vi "Fpga-OrderBook.vi"() -> ()   [LabVIEW 2016]
uses:
  <vilib>/Platform/TimedLoop/XDataNode/timing_clust.ctl
  <vilib>/Platform/TimedLoop/XDataNode/nitl_modes.ctl
  <vilib>/Platform/TimedLoop/XDataNode/wakeup.ctl
  <vilib>/rvi/Emulation/niFpgaSctlEmulationGetInTimedLoop.vi
  <vilib>/rvi/Emulation/niFpgaEmulationReportErrorSimple.vi
  <vilib>/rvi/Emulation/niFpgaGetClockAttributes.vi
  <vilib>/rvi/Emulation/niFpgaCriticalErrorInLSC.vi
  <vilib>/rvi/DataTransferAndStorage/Container/Common/niFpgaContainerGetUniqueNameForEmu.vi
  <vilib>/rvi/DataTransferAndStorage/Container/Common/niFpgaContainerSetEmuInfo.vi
  <vilib>/rvi/eio/common/nirviEmuReportErrorAndStop.vi
  <vilib>/rvi/DataTransferAndStorage/Container/Common/niFpgaContainerExecOnDevCompGetState.vi
  <vilib>/rvi/Emulation/niFpgaEmulationIsFPGAContextNoSignature.vi
  <vilib>/rvi/Emulation/niFpgaProcessEmulError.vi
  <vilib>/rvi/errors/nirviReportUnexpectedCaseInternalError (U32).vi
  <vilib>/rvi/Memory/Memory_Emulation/niFpgaMemoryEmulationCacheClearOnFirstRun.vi
  <vilib>/rvi/Memory/Memory_Emulation/nirvimemoryEmulationManagerCache_MakeExclusive.vi
  <vilib>/rvi/Memory/Memory_Emulation/niFpgaMemoryEmulationValidateCache.vi
  <vilib>/rvi/Memory/Memory_Emulation/nirvimemoryEmulationManagerCache_InsertValue.vi
  <vilib>/Utility/error.llb/Clear Errors.vi
  <vilib>/rvi/Memory/Memory_Emulation/nirvimemoryEmulationManagerCache_ReleaseExclusive.vi
  <vilib>/rvi/Memory/Memory_Emulation/nirvimemoryEmulationManagerCache_GetValue.vi
  <vilib>/rvi/Memory/Memory_Emulation/nirvimemoryEmulationManagerCache_SetValue.vi
  <vilib>/rvi/Emulation/niFpgaSctlEmulationResourceMgr.vi
  <vilib>/rvi/errors/niFpgaSetErrorForExecOnDevCompSimple.vi
  <vilib>/rvi/FIFO/Fifo_Resource/nirvififoEmulationSetSize.vi
  <vilib>/rvi/FIFO/Fifo_Resource/nirviFifoEmulationQueueMgr.vi
  <instcachedir>/0/nirviFifoEmulationQueueMgr_E5CAEC123FF24DC58D834DCA3CDAA9B5.lvgen/nirviFifoEmulationQueueMgr_E5CAEC123FF24DC58D834DCA3CDAA9B5_000.vi
  <vilib>/rvi/FIFO/Fifo_Resource/nirvififoEmulationDetermineInputValidOut.vi
  <vilib>/rvi/FIFO/Fifo_Resource/nirvififoEmulationCreateLock.vi
  <vilib>/rvi/FIFO/Fifo_Resource/nirvififoEmulationObtainLock.vi
  <vilib>/rvi/FIFO/Fifo_Resource/nirvififoEmulationReleaseLock.vi
  <vilib>/rvi/occurrence/nirviWaitOnOccurrenceBase.vi
  <vilib>/rvi/errors/nirviReportUnexpectedCaseInternalError.vi
  <vilib>/Platform/TimedLoop/XDataNode/XDataNode.xnode
  <vilib>/rvi/LocalResourceManager/LocalResourceManager.xnode
  <vilib>/rvi/DataTransferAndStorage/Container/XNode/niFpgaContainer.xnode
  <vilib>/rvi/Memory/Memory_Emulation/niFpgaMemoryEmulationRefIn.vi
  <vilib>/rvi/FIFO/Fifo_Resource/nirvififoEmulationWrite.vi
  <vilib>/rvi/FIFO/Fifo_Resource/nirvififoEmulationRead.vi
  <vilib>/Platform/TimedLoop/XDataNode/XDNodeRunTimeDep.lvlib
panel:
  out "Command being Read":bool
  out "Command":T1 {"OrderRefNum" format="%.0x"}
  out "Command\nExecuting":bool
  out "Counter":u64 format="%.0x"
  out "Command":u16 format="%.0x"
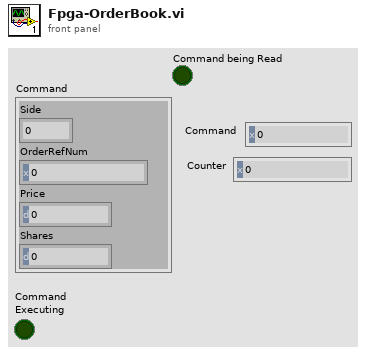
[diagram p1: front panel]
types:
  T1 = cluster{"Side":u16, "OrderRefNum":u64, "Price":u32, "Shares":u32}
  T2 = typedef "XDNodeRunTimeDep.lvlib/timing_clust.ctl" = cluster{"Expected End [f-1]":u64, "Actual End [f-1]":u64, "Finished Late? [f-1]":bool, "Expected End [i-1]":u64, "Actual End [i-1]":u64, "Finished Late? [i-1]":bool, "Expected Start [i]":u64, "Actual Start [i]":u64, "Expected Start [f]":u64, "Actual Start [f]":u64, "Source Name":string, "Structure Name":string, "Period":i64, "Deadline":i64, "Offset":i64, "Start":i64, "Priority":i32, "Timeout":i32, "Mode":T3, "Wakeup Reason":T4, "Error":errorcluster, "Source Type":string, "Secondary Source Type":string, "Global End Time":u64, "Global Start Time":u64, "Frame Duration":u64, "Iteration Duration":u64, "Assigned CPU":i32, "I/O Scan Engine Mode":u32}
  T3 = typedef "XDNodeRunTimeDep.lvlib/nitl_modes.ctl" = enum32{"No Change", "Process missed periods, maintain original phase", "Discard missed periods, maintain original phase", "Process missed periods, ignore original phase", "Discard missed periods, ignore original phase"}
  T4 = typedef "XDNodeRunTimeDep.lvlib/wakeup.ctl" = enum32{"Normal", "Aborted", "Asynchronous wakeup", "Timing source error", "Timed loop error", "Timeout"}
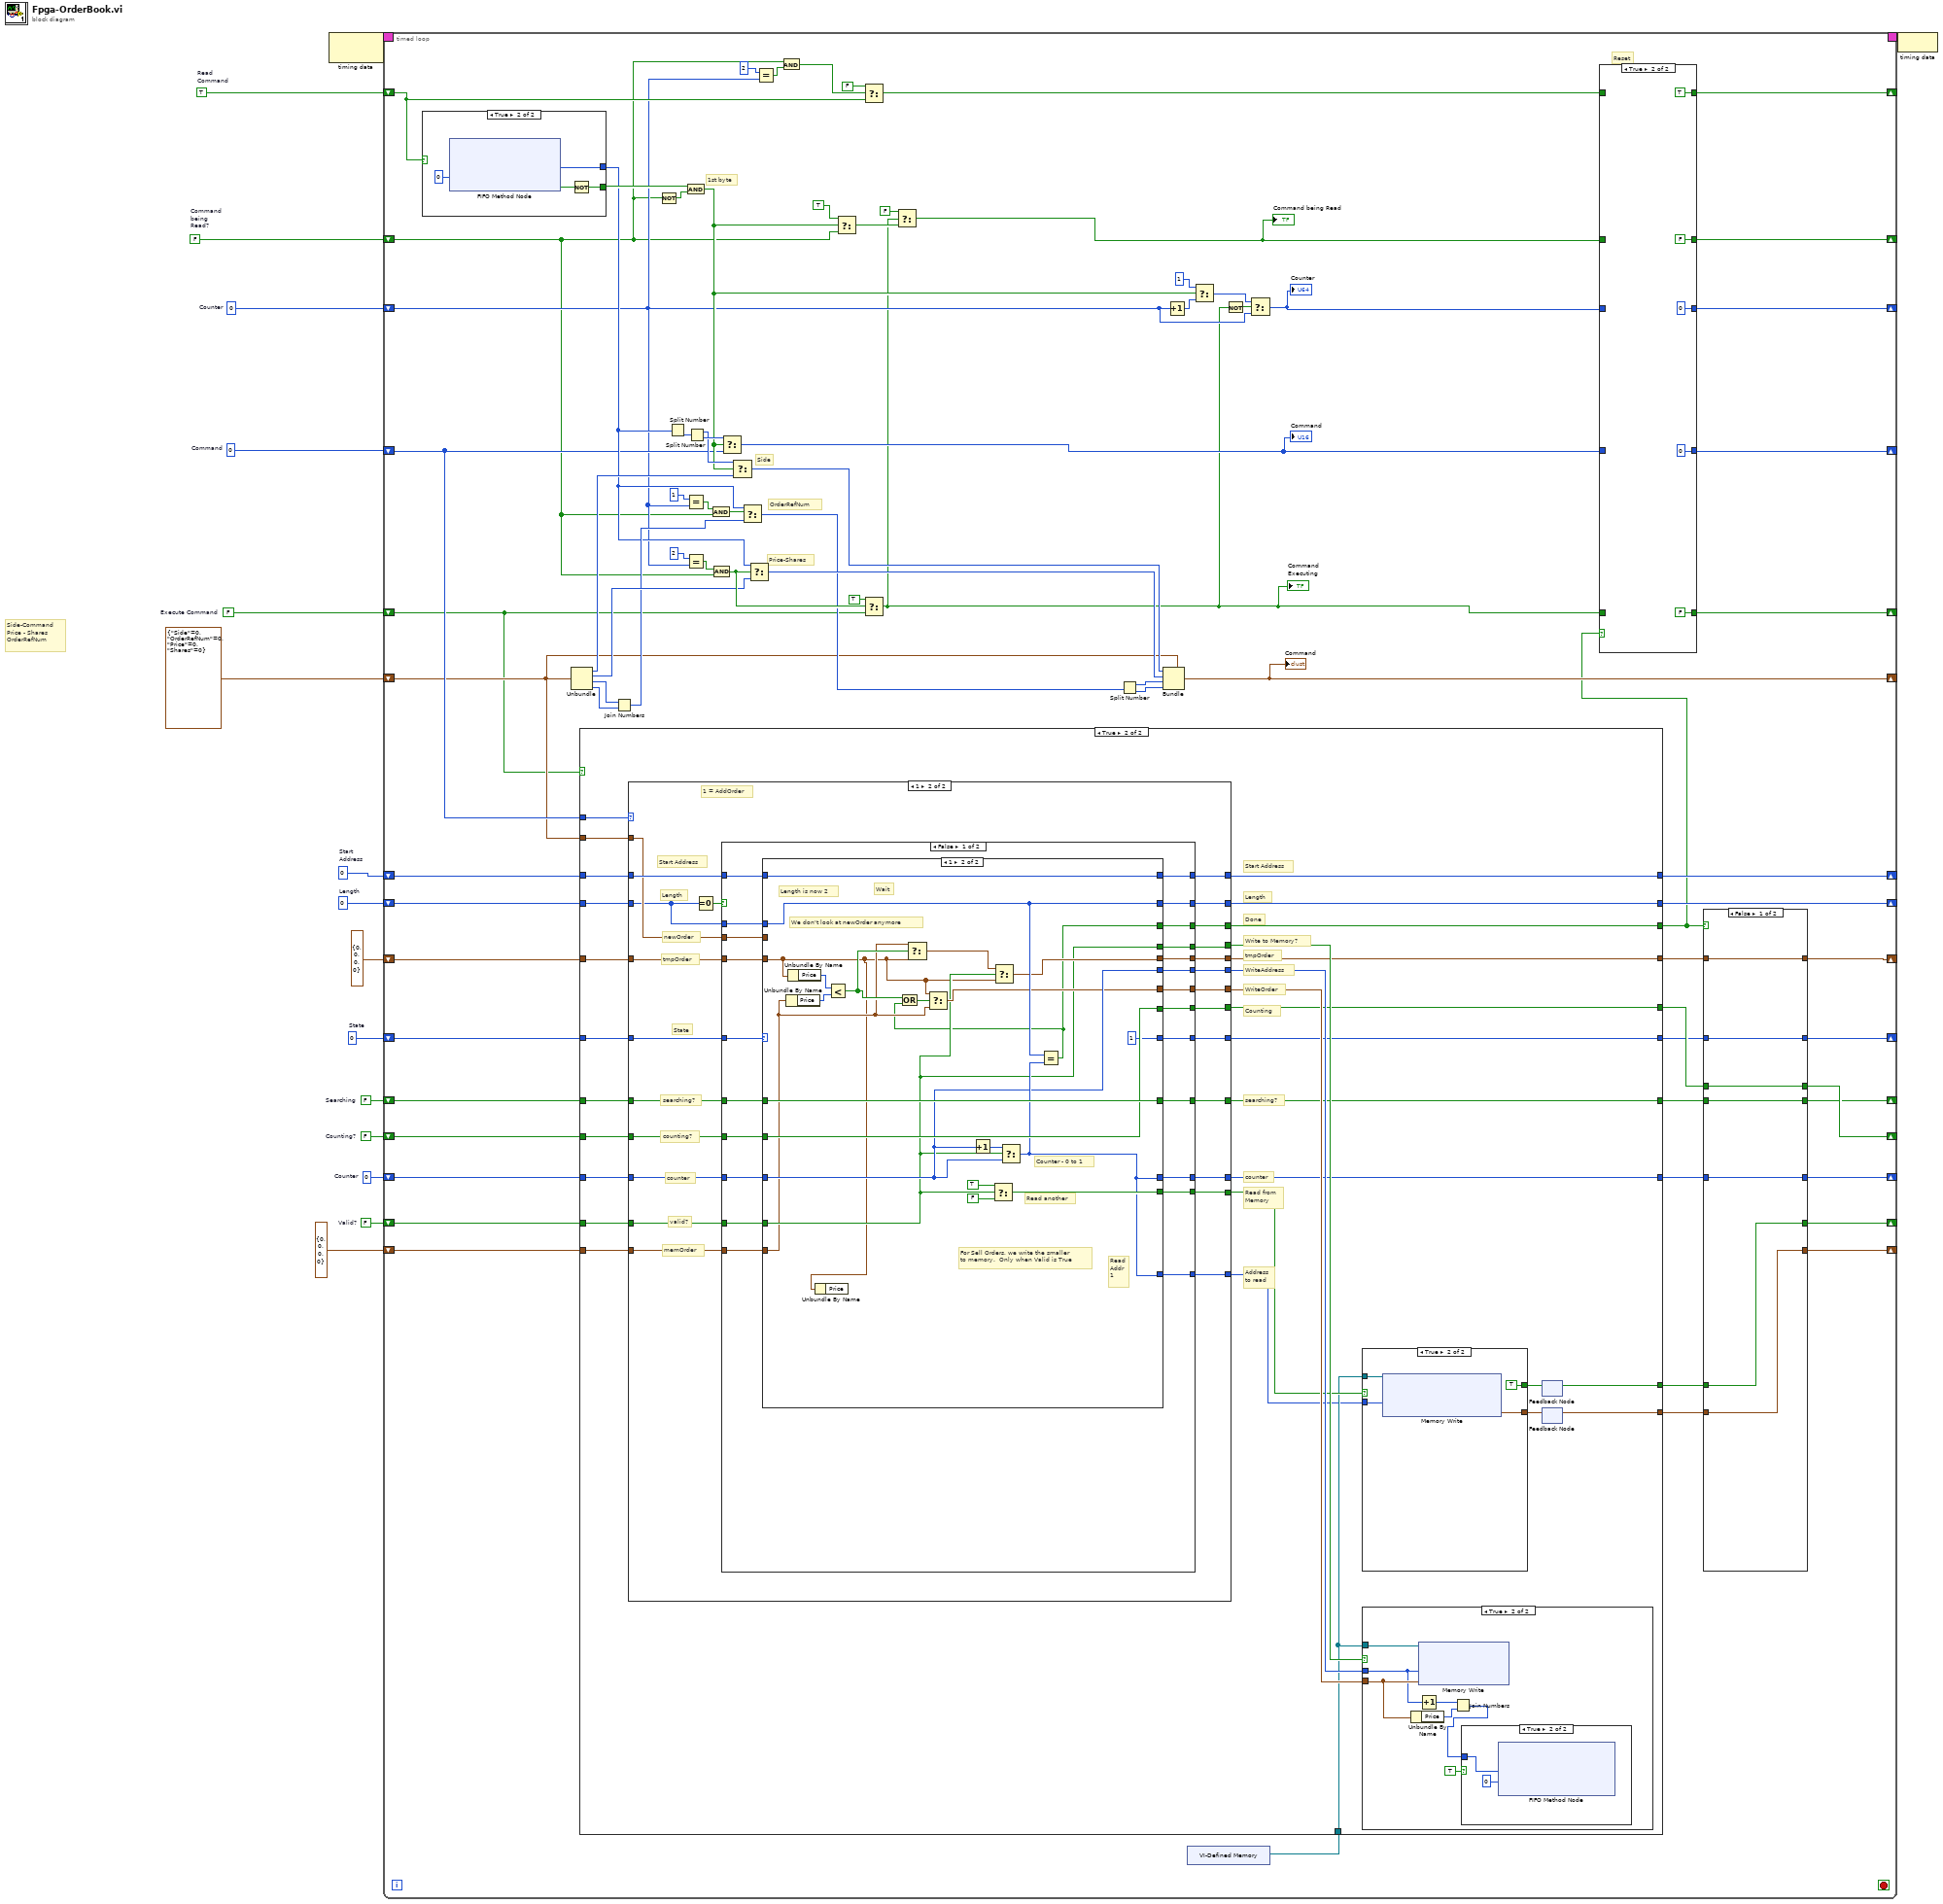
[diagram p0: block diagram]
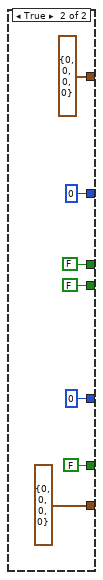
[diagram p2: hidden frame]
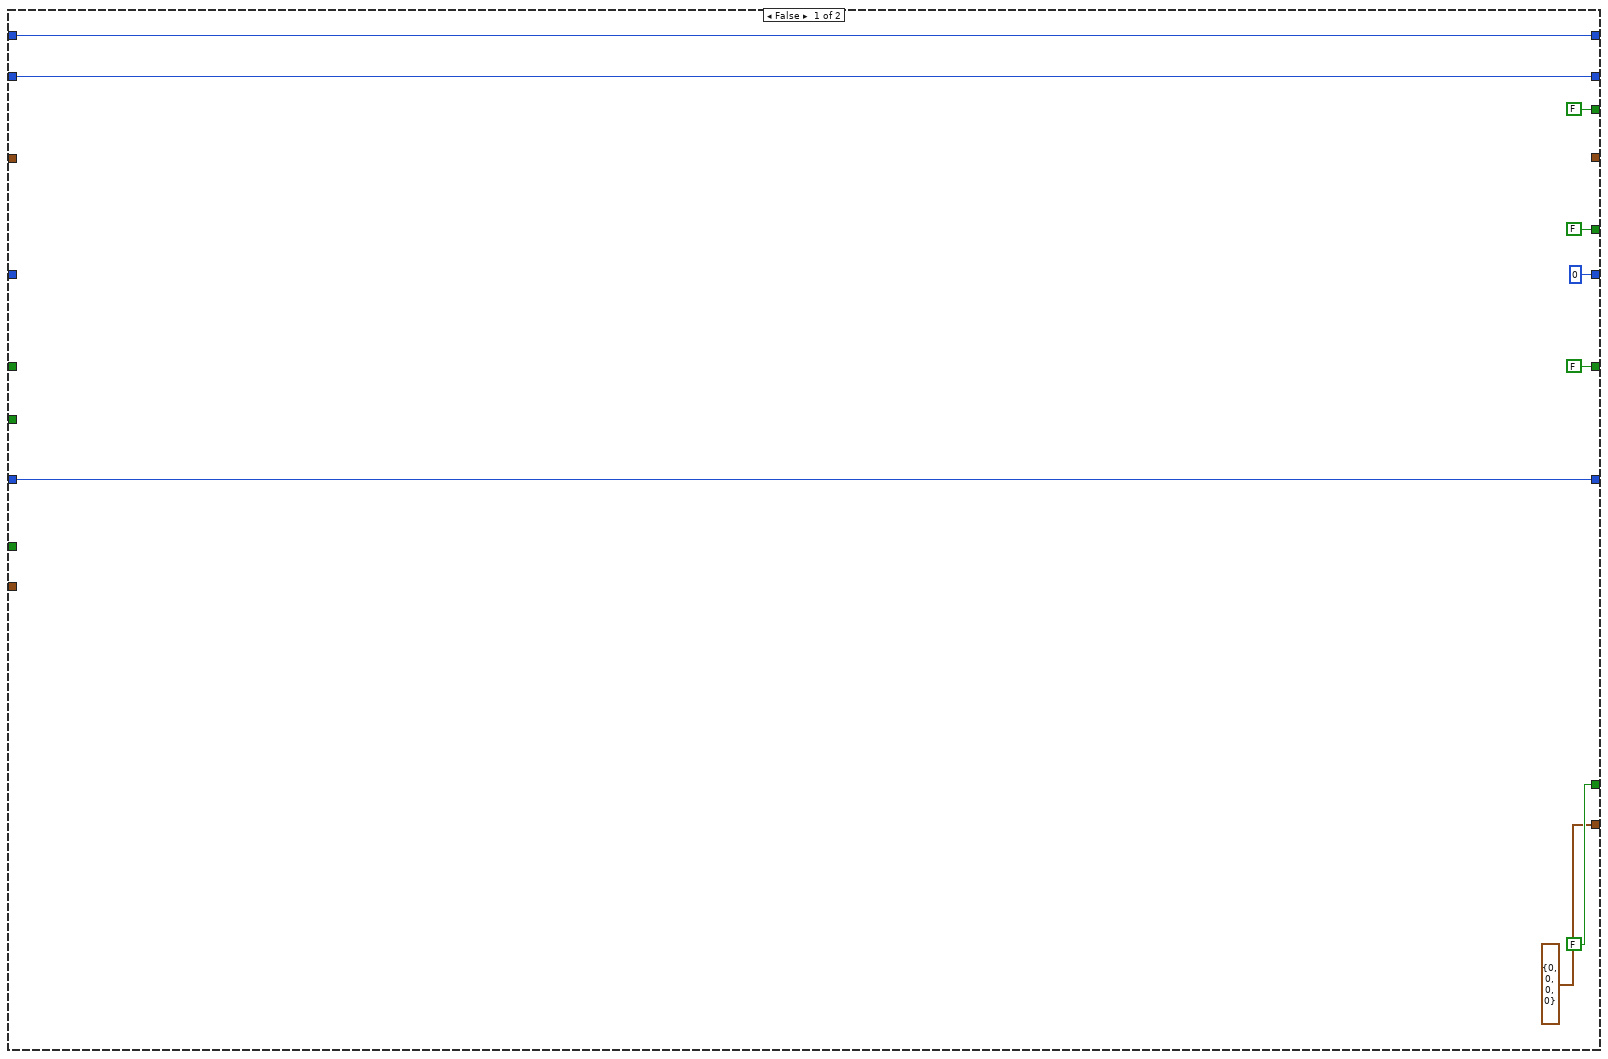
[diagram p4: hidden frame]
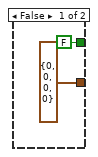
[diagram p5: hidden frame]
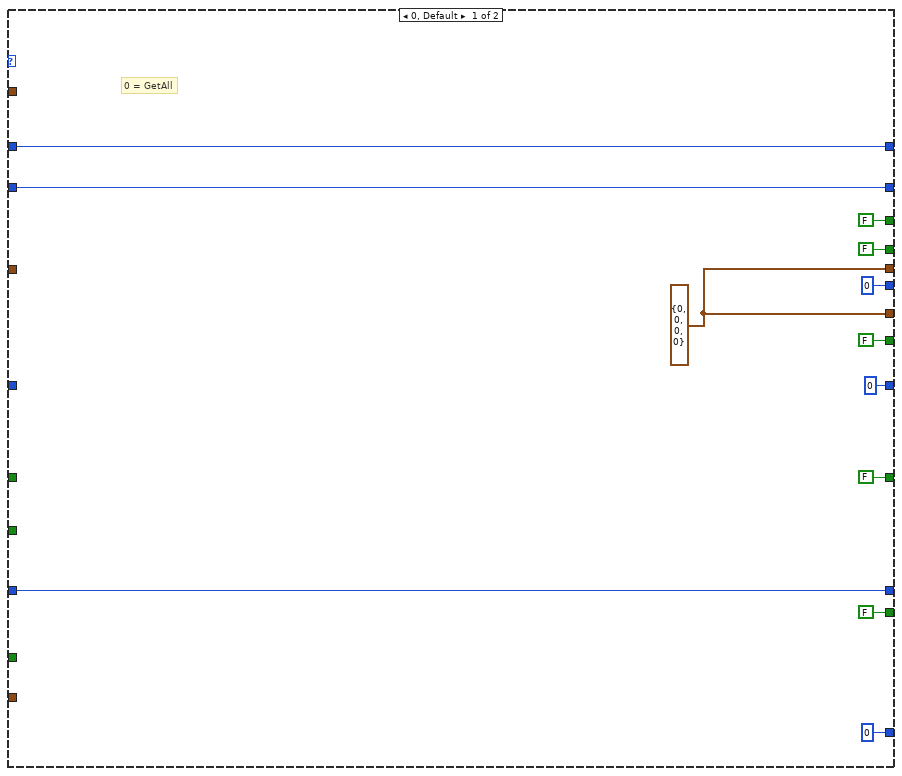
[diagram p8: hidden frame]
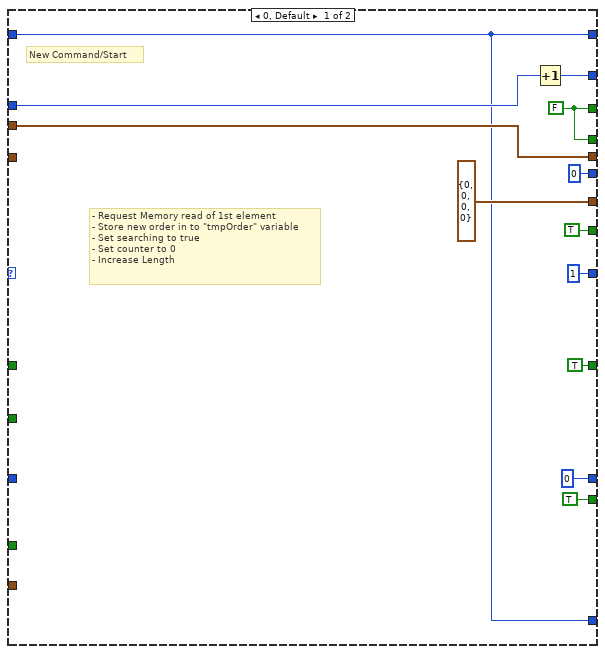
[diagram p9: hidden frame]
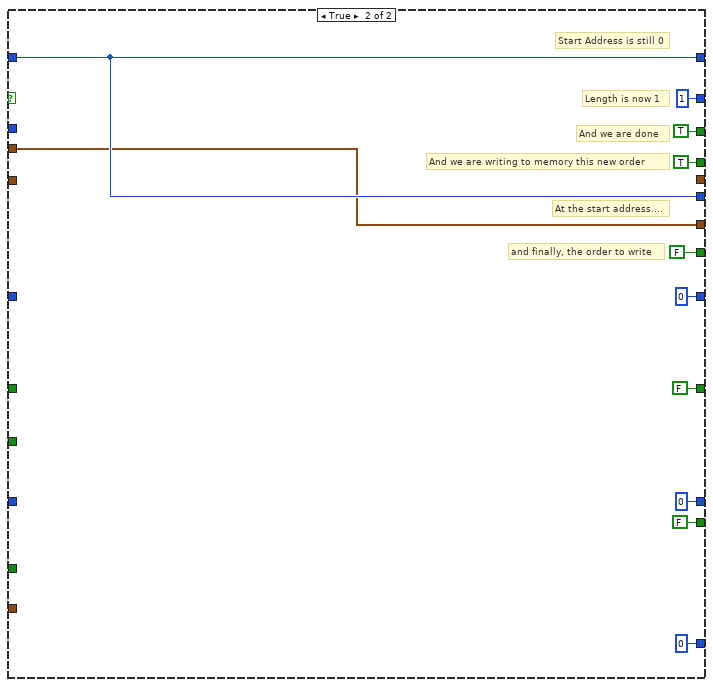
[diagram p10: hidden frame]
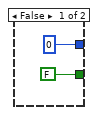
[diagram p11: hidden frame]
diagram:
  w1 = i16 0  # State
  w3 = FALSE  # Searching
  w5 = FALSE  # Valid?
  w6 = FALSE  # Counting?
  w8 = u64 0  # Counter
  w9 = FALSE  # Execute Command
  w11 = u64 0  # Length
  w10 = u64 0  # Start Address
  w12 = u64 0  # Counter
  w13 = u16 0  # Command
  w14 = FALSE  # Command being Read?
  w15 = TRUE  # Read Command
  # "Side-Command\nPrice - Shares\nOrderRefNum"
  n1 = node-c288() -> (w17:T2)  [unwired: 1 in]
  n2 = timed-loop {
    timing: w17 -> [_]
    timing-out: [_] -> w16
    shift-right: [w47] -> _
    shift-left: w15 -> [w93]
    shift-right: [w46] -> _
    shift-left: w14 -> [w51]
    shift-right: [w42] -> _
    shift-left: w13 -> [w58]
    shift-right: [w44] -> _
    shift-left: w12 -> [w55]
    shift-right: [w86] -> _
    shift-left: w10 -> [w87]
    shift-right: [w88] -> _
    shift-left: w11 -> [w89]
    shift-right: [w40] -> _
    shift-left: w9 -> [w49]
    shift-right: [w29] -> _
    shift-left: w8 -> [w79]
    shift-right: [w73] -> _
    shift-left: T1 {"Side"=0, "OrderRefNum"=0, "Price"=0, "Shares"=0} ("Cluster") -> [w50]
    shift-right: [w32] -> _
    shift-left: w6 -> [w38]
    shift-right: [w23] -> _
    shift-left: T1 {"Side"=0, "OrderRefNum"=0, "Price"=0, "Shares"=0} ("Data") -> [w36]
    shift-right: [w24] -> _
    shift-left: w5 -> [w37]
    shift-right: [w31] -> _
    shift-left: w3 -> [w35]
    shift-right: [w27] -> _
    shift-left: T1 {"Side"=0, "OrderRefNum"=0, "Price"=0, "Shares"=0} ("Data") -> [w34]
    shift-right: [w20] -> _
    shift-left: w1 -> [w21]
    stop <- _ stop-if-true
    # "Reset"
    # "Price-Shares"
    # "OrderRefNum"
    # "Side"
    # "1st byte"
    n3 = case shown="True" w93 {
      tunnel: [FALSE ("Timed Out?") w280] -> w95
      tunnel: [u64 0 ("Element") w281] -> w60
      frame False {
      }
      frame True {
        n4 = xnode ("FIFO Method Node")("Timeout"=0) -> ("Element"=w281:u64, "Timed Out?"=w282:bool)  [unwired: 1 in, 1 out]
        n5 = Not(x=w282) -> (.not. x?=w280:bool)
      }
    }
    n6 = Unbundle(w50) -> ("Side"=w63:u16, "OrderRefNum"=w70:u64, "Price"=w66:u32, "Shares"=w65:u32)
    n7 = Join Numbers(hi=w66, lo=w65) -> ((hi.lo)=w61:u64)
    n8 = Not(x=w51) -> (.not. x?=w96:bool)
    n9 = Split Number(x=w60) -> (lo(x)=w72:u32)  [unwired: 1 out]
    n10 = And(x=w95, y=w96) -> (x .and. y?=w59:bool)
    n11 = Equal?(x=u64 1, y=w55) -> (x = y?=w52:bool)
    n12 = Equal?(x=u64 2, y=w55) -> (x = y?=w77:bool)
    n13 = Split Number(x=w72) -> (hi(x)=w62:u16, lo(x)=w64:u16)
    n14 = And(x=w52, y=w51) -> (x .and. y?=w53:bool)
    n15 = And(x=w77, y=w51) -> (x .and. y?=w78:bool)
    n16 = Select(t=w64, s=w59, f=w58) -> (s? t:f=w41:u16)
    "Command" <- w41
    n17 = Select(t=w62, s=w59, f=w63) -> (s? t:f=w57:u16)
    n18 = Select(t=w60, s=w53, f=w61) -> (s? t:f=w69:u64)
    n19 = Select(t=w60, s=w78, f=w70) -> (s? t:f=w71:u64)
    n20 = Equal?(x=u64 2, y=w55) -> (x = y?=w82:bool)
    n21 = And(x=w51, y=w82) -> (x .and. y?=w84:bool)
    n22 = Select(t=TRUE, s=w59, f=w51) -> (s? t:f=w75:bool)
    n23 = Select(t=FALSE, s=w84, f=w93) -> (s? t:f=w48:bool)
    n24 = Select(t=TRUE, s=w78, f=w49) -> (s? t:f=w39:bool)
    "Command\nExecuting" <- w39
    n25 = Select(t=FALSE, s=w39, f=w75) -> (s? t:f=w45:bool)
    "Command being Read" <- w45
    n26 = Split Number(x=w69) -> (hi(x)=w68:u32, lo(x)=w67:u32)
    n27 = Bundle(cluster=w50, "Side"=w57, "OrderRefNum"=w71, "Price"=w68, "Shares"=w67) -> (w73:T1)
    "Command" <- w73
    n28 = Increment(x=w55) -> (x+1=w91:u64)
    n29 = xnode "VI-Defined Memory"() -> ("Memory Out"=w74:refnum<k21>)
    n30 = case shown="True" w49 {
      tunnel: w58 -> [_ w158]
      tunnel: w89 -> [w129 w157]
      tunnel: [w129 w156] -> w88
      tunnel: w87 -> [w128 w154]
      tunnel: [w128 w155] -> w86
      tunnel: w79 -> [w126 w153]
      tunnel: [w126 w144] -> w28
      tunnel: [FALSE w152] -> w25
      tunnel: w74 -> [_ w145]
      tunnel: w50 -> [_ w139]
      tunnel: w38 -> [_ w148]
      tunnel: [FALSE w147] -> w33
      tunnel: [T1 {"Side"=0, "OrderRefNum"=0, "Price"=0, "Shares"=0} ("Data") w130] -> w22
      tunnel: [FALSE w131] -> w18
      tunnel: w37 -> [_ w141]
      tunnel: w36 -> [_ w140]
      tunnel: w35 -> [_ w138]
      tunnel: [FALSE w137] -> w30
      tunnel: w34 -> [_ w135]
      tunnel: [_ w134] -> w26
      tunnel: w21 -> [_ w133]
      tunnel: [i16 0 ("State") w132] -> w19
      frame False {
      }
      frame True {
        # "tmpOrder"
        # "searching?"
        # "counter"
        # "Read from\nMemory"
        # "Address\nto read"
        # "Counting"
        # "WriteOrder"
        # "WriteAddress"
        # "Write to Memory?"
        # "Length"
        # "Start Address"
        # "Done"
        n31 = case shown="1" w158 {
          tunnel: w157 -> [w185 w187]
          tunnel: [w185 w209] -> w156
          tunnel: [w184 w207] -> w155
          tunnel: w154 -> [w184 w206]
          tunnel: w153 -> [w183 w198]
          tunnel: [w183 w197] -> w144
          tunnel: [FALSE w205] -> w152
          tunnel: [FALSE w204] -> w151
          tunnel: w139 -> [_ w202]
          tunnel: [w175 w201] -> w150
          tunnel: [u64 0 ("Start\nAddress") w203] -> w149
          tunnel: w148 -> [_ w200]
          tunnel: [FALSE ("Counting?") w199] -> w147
          tunnel: [FALSE ("t") w193] -> w146
          tunnel: w141 -> [_ w192]
          tunnel: w140 -> [_ w191]
          tunnel: w138 -> [_ w196]
          tunnel: [FALSE w195] -> w137
          tunnel: [u64 0 w194] -> w136
          tunnel: w135 -> [_ w190]
          tunnel: [w175 w189] -> w134
          tunnel: w133 -> [_ w188]
          tunnel: [i16 0 ("State") w186] -> w132
          frame 0, Default {
            w175 = T1 {"Side"=0, "OrderRefNum"=0, "Price"=0, "Shares"=0} ("Cluster")
            # "0 = GetAll"
          }
          frame 1 {
            # "State"
            # "Length"
            # "Start Address"
            # "memOrder"
            # "valid?"
            # "counter"
            # "counting?"
            # "searching?"
            # "tmpOrder"
            # "newOrder"
            # "1 = AddOrder"
            n32 = Equal To 0?(x=w187) -> (x = 0?=w208:bool)
            n33 = case shown="False" w208 {
              tunnel: [w231 u64 1 ("t")] -> w209
              tunnel: [w220 w274] -> w207
              tunnel: w206 -> [w219 w274]
              tunnel: [w227 TRUE] -> w205
              tunnel: [w226 TRUE] -> w204
              tunnel: [w225 w274] -> w203
              tunnel: w202 -> [w228 w273]
              tunnel: [w229 w273] -> w201
              tunnel: w200 -> [w210 _]
              tunnel: [w223 FALSE] -> w199
              tunnel: w198 -> [w212 _]
              tunnel: [w217 u64 0] -> w197
              tunnel: w196 -> [w211 _]
              tunnel: [w222 FALSE] -> w195
              tunnel: [w218 u64 0] -> w194
              tunnel: [w221 FALSE] -> w193
              tunnel: w192 -> [w215 _]
              tunnel: w191 -> [w213 _]
              tunnel: w190 -> [w214 _]
              tunnel: [w224 _] -> w189
              tunnel: w188 -> [w232 _]
              tunnel: w187 -> [w230 _]
              tunnel: [w216 i16 0 ("State")] -> w186
              frame False {
                n34 = case shown="1" w232 {
                  tunnel: [w233 w257] -> w231
                  tunnel: w230 -> [w244 w257]
                  tunnel: [T1 {"Side"=0, "OrderRefNum"=0, "Price"=0, "Shares"=0} ("Cluster") w253] -> w229
                  tunnel: w228 -> [w241 _]
                  tunnel: [w243 w245] -> w227
                  tunnel: [w243 w249] -> w226
                  tunnel: [u64 0 ("Start\nAddress") w256] -> w225
                  tunnel: [w241 w252] -> w224
                  tunnel: [TRUE w264] -> w223
                  tunnel: [TRUE w265] -> w222
                  tunnel: [TRUE w263] -> w221
                  tunnel: [w236 w266] -> w220
                  tunnel: w219 -> [w236 w266]
                  tunnel: [w236 w258] -> w218
                  tunnel: [u64 0 w258] -> w217
                  tunnel: [i16 1 ("State") i16 1 ("State")] -> w216
                  tunnel: w215 -> [_ w249]
                  tunnel: w214 -> [_ w246]
                  tunnel: w213 -> [_ w247]
                  tunnel: w212 -> [_ w256]
                  tunnel: w211 -> [_ w265]
                  tunnel: w210 -> [_ w264]
                  frame 0, Default {
                    w243 = FALSE
                    # "- Request Memory read of 1st element\n- Store new order in to \"tmpOrder\" variable\n- Set searching to true\n- Set counter to 0\n- Increase Length"
                    # "New Command/Start"
                    n35 = Increment(x=w244) -> (x+1=w233:u64)
                  }
                  frame 1 {
                    # "Read\nAddr\n1"
                    # "Read another"
                    # "Counter - 0 to 1"
                    # "Wait"
                    # "For Sell Orders, we write the smaller\nto memory.  Only when Valid is True"
                    # "We don't look at newOrder anymore"
                    # "Length is now 2"
                    n36 = Unbundle By Name(w247) -> ("Price"=w254:u32)
                    n37 = Unbundle By Name(w246) -> ("Price"=w255:u32)
                    n38 = Unbundle By Name(w246) -> ()  [unwired: 1 out]
                    n39 = Less?(x=w255, y=w254) -> (x < y?=w250:bool)
                    n40 = Select(t=w247, s=w250, f=w246) -> (s? t:f=w251:T1)
                    n41 = Increment(x=w256) -> (x+1=w260:u64)
                    n42 = Select(t=TRUE, s=w249, f=FALSE) -> (s? t:f=w263:bool)
                    n43 = Select(t=w251, s=w249, f=w246) -> (s? t:f=w252:T1)
                    n44 = Select(t=w260, s=w249, f=w256) -> (s? t:f=w258:u64)
                    n45 = Equal?(x=w257, y=w258) -> (x = y?=w245:bool)
                    n46 = Or(x=w250, y=w245) -> (x .or. y?=w248:bool)
                    n47 = Select(t=w246, s=w248, f=w247) -> (s? t:f=w253:T1)
                  }
                }
              }
              frame True {
                # "and finally, the order to write"
                # "At the start address...."
                # "And we are writing to memory this new order"
                # "And we are done"
                # "Length is now 1"
                # "Start Address is still 0"
              }
            }
          }
        }
        n48 = case shown="True" w146 {
          tunnel: w145 -> [_ w164]
          tunnel: w136 -> [_ w163]
          tunnel: [T1 {"Side"=0, "OrderRefNum"=0, "Price"=0, "Shares"=0} ("Data") w162] -> w143
          tunnel: [FALSE TRUE] -> w142
          frame False {
          }
          frame True {
            n49 = xnode ("Memory Write")("Address"=w163, "Memory In"=w164) -> ("Data"=w162:T1)  [unwired: 1 out]
          }
        }
        n50 = case shown="True" w151 {
          tunnel: w145 -> [_ w171]
          tunnel: w150 -> [_ w170]
          tunnel: w149 -> [_ w169]
          frame False {
          }
          frame True {
            n51 = Unbundle By Name(w170) -> ("Price"=w168:u32)
            n52 = xnode ("Memory Write")("Address"=w169, "Data"=w170, "Memory In"=w171) -> ()  [unwired: 1 out]
            n53 = Increment(x=w169) -> (x+1=w167:u64)
            n54 = Join Numbers(hi=w167, lo=w168) -> ((hi.lo)=w166:u64)
            n55 = case shown="True" TRUE {
              tunnel: w166 -> [_ w172]
              frame False {
              }
              frame True {
                n56 = xnode ("FIFO Method Node")("Element"=w172, "Timeout"=0) -> ()  [unwired: 1 in, 2 out]
              }
            }
          }
        }
        n57 = feedback-in #1(w142) -> ()
        n58 = feedback #1() -> (w131:bool)  [unwired: 1 in]
        n59 = feedback-in #2(w143) -> ()
        n60 = feedback #2() -> (w130:T1)  [unwired: 1 in]
      }
    }
    n61 = Select(t=u64 1, s=w59, f=w91) -> (s? t:f=w54:u64)
    n62 = Not(x=w39) -> (.not. x?=w56:bool)
    n63 = Select(t=w54, s=w56, f=w55) -> (s? t:f=w43:u64)
    "Counter" <- w43
    n64 = case shown="True" w25 {
      tunnel: w48 -> [w115 _]
      tunnel: [w115 TRUE ("Read\nCommand")] -> w47
      tunnel: [w114 FALSE ("Command\nbeing\nRead?")] -> w46
      tunnel: w45 -> [w114 _]
      tunnel: [w113 u64 0 ("Counter")] -> w44
      tunnel: w43 -> [w113 _]
      tunnel: [w112 u16 0 ("Command")] -> w42
      tunnel: w41 -> [w112 _]
      tunnel: [w111 FALSE ("Execute Command")] -> w40
      tunnel: w39 -> [w111 _]
      frame False {
      }
      frame True {
      }
    }
    n65 = case shown="False" w25 {
      tunnel: w33 -> [w103 _]
      tunnel: [w103 FALSE ("Counting?")] -> w32
      tunnel: [w102 FALSE] -> w31
      tunnel: w30 -> [w102 _]
      tunnel: [w101 u64 0 ("Counter")] -> w29
      tunnel: w28 -> [w101 _]
      tunnel: [w100 T1 {"Side"=0, "OrderRefNum"=0, "Price"=0, "Shares"=0} ("Cluster")] -> w27
      tunnel: w26 -> [w100 _]
      tunnel: [w99 FALSE] -> w24
      tunnel: w18 -> [w99 _]
      tunnel: [w98 T1 {"Side"=0, "OrderRefNum"=0, "Price"=0, "Shares"=0} ("Data")] -> w23
      tunnel: w22 -> [w98 _]
      tunnel: [w97 i16 0 ("State")] -> w20
      tunnel: w19 -> [w97 _]
      frame False {
      }
      frame True {
      }
    }
  }
  n66 = node-c288(w16) -> ()
